vi "PKG_IMC_GetConfig.vi"(0 "handle":u32, 1 "steptime":i32, 2 "pulpolar":i32, 3 "dirpolar":i32, 4 "encpena":i32, 5 "encpmode":i32, 6 "encpdir":i32, 8 "vellim":dbl, 9 "acclim":dbl, 10 "drvena":i32, 11 "plimena":i32, 12 "plimpolar":i32, 13 "nlimena":i32, 14 "nlimpolar":i32, 15 "almena":i32, 16 "almpolar":i32, 17 "INPena":i32, 18 "INPpolar":i32, 19 "axis":i32) -> (20 "handle out":u32, 21 "steptime out":i32, 22 "pulpolar out":i32, 23 "dirpolar out":i32, 24 "encpena out":i32, 25 "encpmode out":i32, 26 "encpdir out":i32)   [LabVIEW 2011, in "IMC_Pkg4xxx.lvlib"]
doc: "PKG_IMC_GetConfig(IMC_HANDLE handle, int *steptime, int *pulpolar, int *dirpolar, int *encpena, int *encpmode, int *encpdir, double *vellim, double *acclim, int *drvena, int *plimena, int *plimpolar, int *nlimena, int *nlimpolar, int *almena, int *almpolar, int *INPena, int *INPpolar, int axis);"
uses:
  IMC_Pkg4xxx.lvlib
  IMC_Pkg4xxx.dll
panel:
  out "INPpolar out":i32
  out "INPena out":i32
  out "almpolar out":i32
  out "almena out":i32
  out "nlimpolar out":i32
  out "nlimena out":i32
  out "plimpolar out":i32
  out "plimena out":i32
  out "drvena out":i32
  out "acclim out":dbl
  out "vellim out":dbl
  out "function return":i32
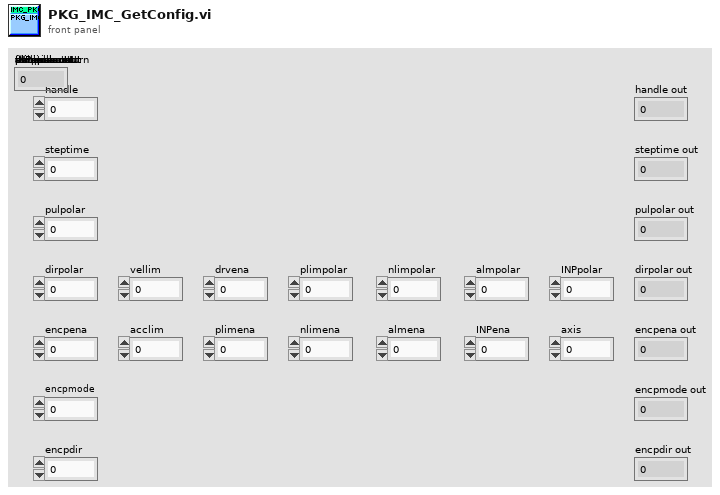
[diagram p1: front panel]
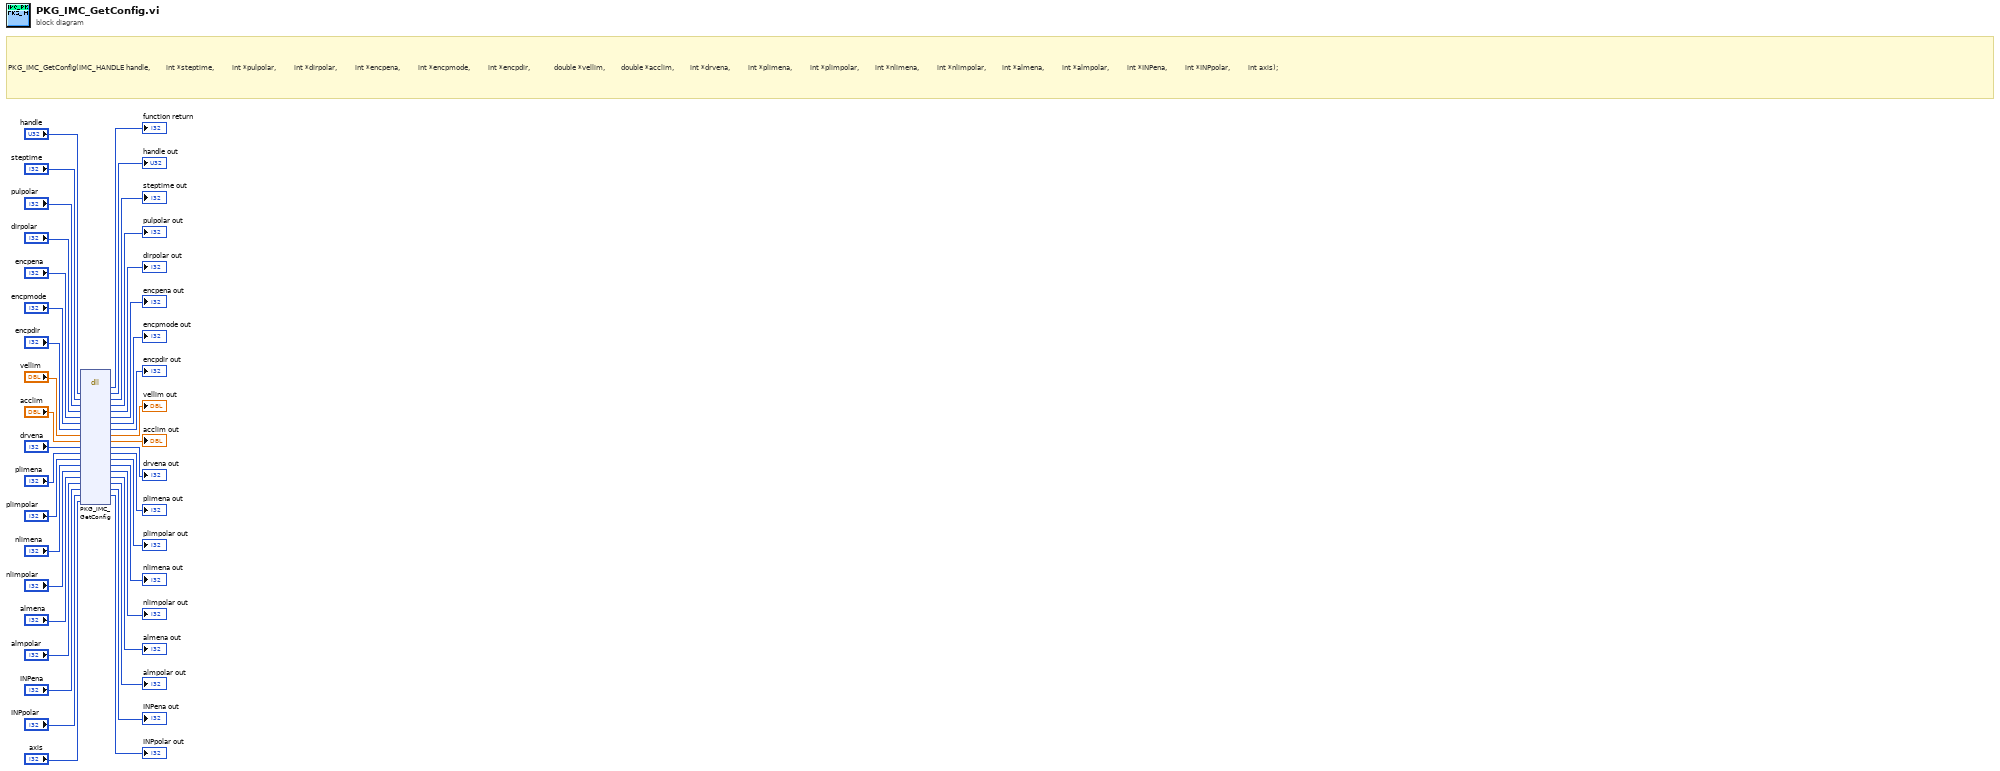
[diagram p0: block diagram]
diagram:
  # "PKG_IMC_GetConfig(IMC_HANDLE handle,  \t\t\t\t\t\tint *steptime, \t\t\t\t\t\t\t\tint *pulpolar, \t\t\t\t\t\t\t\tint *dirpolar, \t\t\t\t\t\t\t\tint *encpena, \t\t\t\t\t\t\t\tint *encpmode, \t\t\t\t\t\t\t\tint *encpdir, \t\t\t\t\t\t\t\t\t\t\tdouble *vellim, \t\t\t\t\t\t\tdouble *acclim, \t\t\t\t\t\t\tint *drvena, \t\t\t\t\t\t\t\tint *plimena, \t\t\t\t\t\t\t\tint *plimpolar, \t\t\t\t\t\t\tint *nlimena, \t\t\t\t\t\t\t\tint *nlimpolar, \t\t\t\t\t\t\tint *almena, \t\t\t\t\t\t\t\tint *almpolar, \t\t\t\t\t\t\t\tint *INPena, \t\t\t\t\t\t\t\tint *INPpolar, \t\t\t\t\t\t\t\tint axis);"
  n1 = dll-call lib="PTH1mabs F光盘刻录\niMC MotionIMCNet_V4.0IMCAppincLabviewIMC_PKG4xxxIMC_PKG4xxx\nIMC_Pkg4xxx.*" fn="PKG_IMC_GetConfig"("handle"="handle", "steptime"="steptime", "pulpolar"="pulpolar", "dirpolar"="dirpolar", "encpena"="encpena", "encpmode"="encpmode", "encpdir"="encpdir", "vellim"="vellim", "acclim"="acclim", "drvena"="drvena", "plimena"="plimena", "plimpolar"="plimpolar", "nlimena"="nlimena", "nlimpolar"="nlimpolar", "almena"="almena", "almpolar"="almpolar", "INPena"="INPena", "INPpolar"="INPpolar", "axis"="axis") -> (→"function return":i32, "handle"=→"handle out":u32, "steptime"=→"steptime out":i32, "pulpolar"=→"pulpolar out":i32, "dirpolar"=→"dirpolar out":i32, "encpena"=→"encpena out":i32, "encpmode"=→"encpmode out":i32, "encpdir"=→"encpdir out":i32, "vellim"=→"vellim out":dbl, "acclim"=→"acclim out":dbl, "drvena"=→"drvena out":i32, "plimena"=→"plimena out":i32, "plimpolar"=→"plimpolar out":i32, "nlimena"=→"nlimena out":i32, "nlimpolar"=→"nlimpolar out":i32, "almena"=→"almena out":i32, "almpolar"=→"almpolar out":i32, "INPena"=→"INPena out":i32, "INPpolar"=→"INPpolar out":i32)  [unwired: 4 in, 2 out]
